vi "Prune.vi"(8 "error in (no error)":errorcluster, 10 "Master Device in":refnum<class "Master Device.lvclass">, 11 "Aerotech_Soloist in":refnum<class "Aerotech_Soloist.lvclass">) -> (0 "error out":errorcluster, 2 "Master Device out":refnum<class "Master Device.lvclass">, 3 "Aerotech_Soloist out":refnum<class "Aerotech_Soloist.lvclass">)   [LabVIEW 2013, in "Aerotech_Soloist.lvclass"]
doc: "Prune.vi is the first of two subVIs called in FinalizeHWI. Triggered slave devices need to:\n (1) Re-check triggering from Master Device's \"Slave Info\" to see what ramps are required to be programmed\n (2) Prune those lines from the \"prepared\" image (in reversed order just like triggering and the Ramp List) that will not be triggered.\n\nThe next subVI called is BuildHWI where you will actually flatten the \"prepared\" image and put it in normal time order."
uses:
  Aerotech_Soloist.lvclass
  Master Device/Master Device.lvclass
  Aerotech_Soloist.lvclass/Aerotech_Soloist.ctl
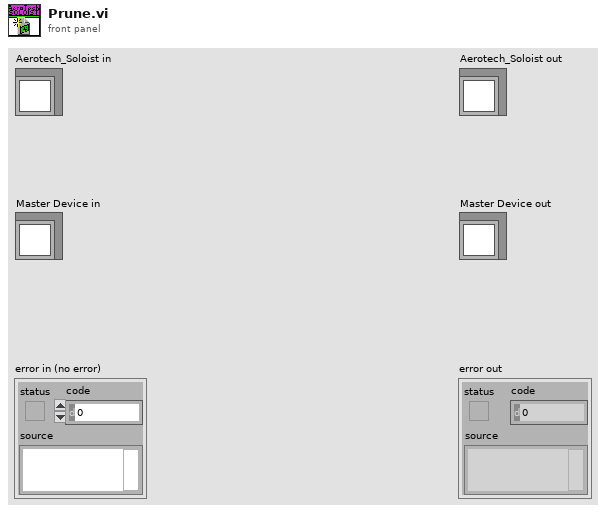
[diagram p1: front panel]
types:
  T1 = typedef "Aerotech_Soloist.lvclass/ParsedSWILine.ctl" = cluster{"ParameterScript":string, "CommandScript":string}
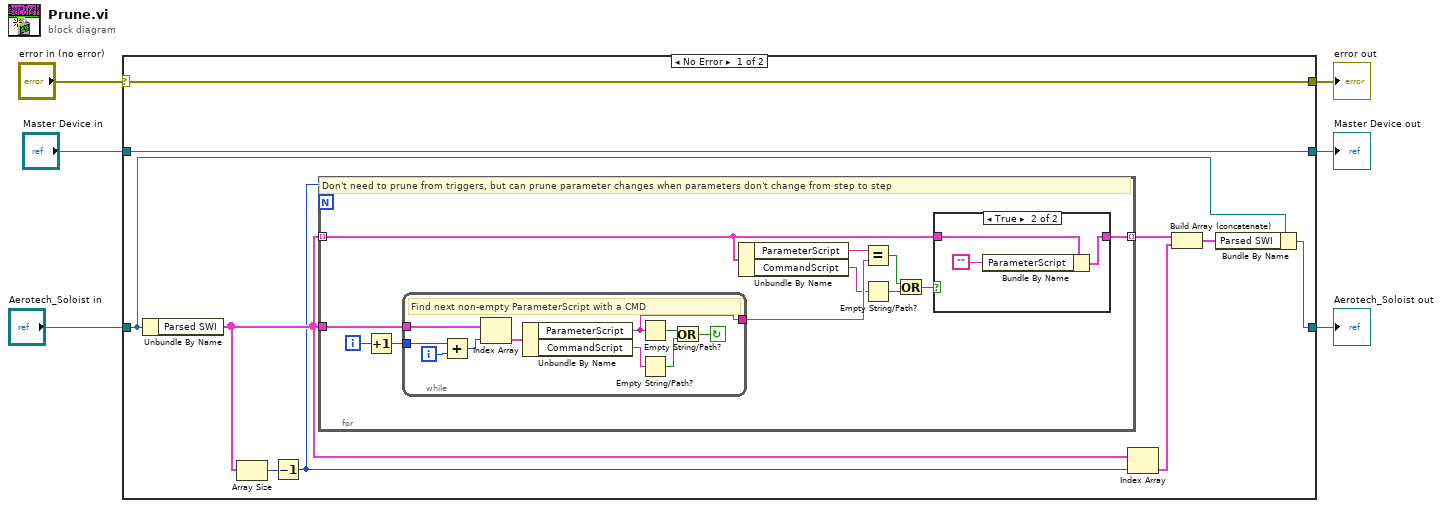
[diagram p0: block diagram]
diagram:
  n1 = case shown="No Error" "error in (no error)" {
    selector: "error in (no error)" -> [w7 w42]
    tunnel: "Aerotech_Soloist in" -> [w10 w43]
    tunnel: [w9 w43] -> w4
    tunnel: [w8 w44] -> w3
    tunnel: "Master Device in" -> [w8 w44]
    tunnel: [w7 w42] -> w1
    frame No Error {
      n2 = Unbundle By Name(w10) -> ("Parsed SWI"=w15:T1[])
      n3 = Array Size(array=w15) -> (size(s)=w16:i32)
      n4 = Decrement(x=w16) -> (x-1=w14:i32)
      n5 = for {
        N: w14 -> [_]
        tunnel: w15 -> [w22]
        tunnel: w15 -> [w25] mode=indexing
        tunnel: [w24] -> w13 mode=indexing
        i -> [w27]
        # "Don't need to prune from triggers, but can prune parameter changes when parameters don't change from step to step"
        n6 = Increment(x=w27) -> (x+1=w23:i32)
        n7 = while {
          tunnel: w23 -> [w35]
          tunnel: w22 -> [w34]
          tunnel: [w32] -> w21
          i -> [w36]
          stop <- w28 continue-if-true
          # "Find next non-empty ParameterScript with a CMD"
          n8 = Add(x=w35, y=w36) -> (x+y=w37:i32)
          n9 = Index Array(array=w34, index=w37) -> (element=w33:T1)
          n10 = Unbundle By Name(w33) -> ("ParameterScript"=w32:string, "CommandScript"=w31:string)
          n11 = Empty String/Path?(string/path=w32) -> (empty?=w29:bool)
          n12 = Empty String/Path?(string/path=w31) -> (empty?=w30:bool)
          n13 = Or(x=w29, y=w30) -> (x .or. y?=w28:bool)
        }
        n14 = Unbundle By Name(w25) -> ("ParameterScript"=w26:string, "CommandScript"=w20:string)
        n15 = Equal?(x=w26, y=w21) -> (x = y?=w17:bool)
        n16 = Empty String/Path?(string/path=w20) -> (empty?=w19:bool)
        n17 = Or(x=w17, y=w19) -> (x .or. y?=w18:bool)
        n18 = case shown="True" w18 {
          tunnel: [w38 w40] -> w24
          tunnel: w25 -> [w38 w41]
          frame False {
          }
          frame True {
            n19 = Bundle By Name(cluster=w41, "ParameterScript"="") -> (w40:T1)
          }
        }
      }
      n20 = Index Array(array=w15, index=w14) -> (element=w12:T1)
      n21 = Build Array (concatenate)(w13, w12) -> (w11:T1[])
      n22 = Bundle By Name(cluster=w10, "Parsed SWI"=w11) -> (w9:refnum<class "Aerotech_Soloist.lvclass">)
    }
    frame Error {
    }
  }
  "error out" <- w1
  "Aerotech_Soloist out" <- w4
  "Master Device out" <- w3
